vi "HMP_Open_v1.vi"(11 "HMP VISA":refnum<visa-resource-name>="HMP") -> (3 "HMP VISA Out":refnum<visa-resource-name>)   [LabVIEW 2019]
panel:
  out "Loop Error?":errorcluster
  in  "stop":bool
  out "Instructional Message":string
  out "Unsuccesful Attempts to connect":i32
  in  "Error In":errorcluster caption="error in (no error)"
  out "Error Out":errorcluster caption="error out"
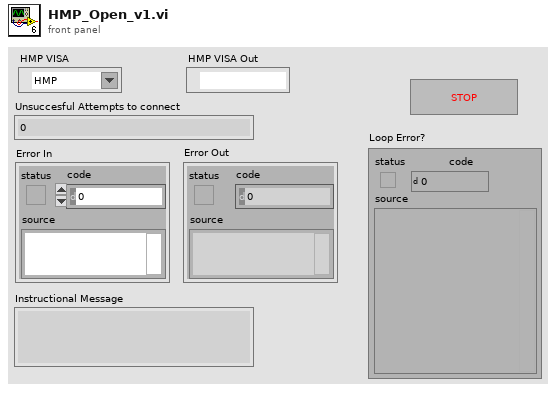
[diagram p1: front panel]
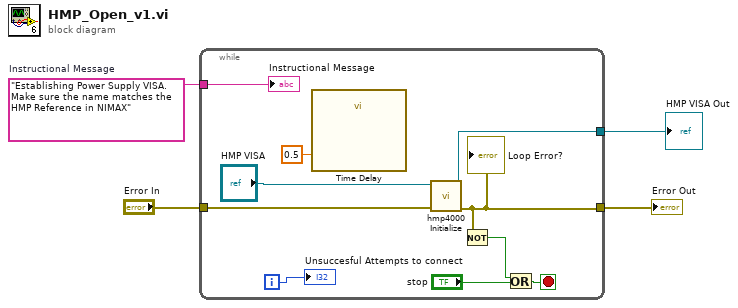
[diagram p0: block diagram]
diagram:
  w2 = "Establishing Power Supply VISA. Make sure the name matches the HMP Reference in NIMAX"  # Instructional Message
  n1 = while {
    tunnel: "Error In" -> [w14]
    tunnel: [w11] -> w4
    tunnel: w2 -> [w9]
    tunnel: [w7] -> w1
    i -> [w8]
    stop <- w10 stop-if-true
    n2 = call "Time Delay"("Delay Time (s)"=0.5) -> ()  [unwired: 10 in, 1 out]
    n3 = call <instrlib>:"hmp4000 Initialize.vi"("error in (no error)"=w14, "VISA resource name"="HMP VISA") -> ("error out"=w11:errorcluster, "VISA resource name out"=w7:refnum<visa-resource-name>)  [unwired: 8 in]
    "Loop Error?" <- w11
    n4 = Not(x=w11) -> (.not. x?=w12:bool)
    n5 = Or(x=w12, y="stop") -> (x .or. y?=w10:bool)
    "Instructional Message" <- w9
    "Unsuccesful Attempts to connect" <- w8
  }
  "Error Out" <- w4
  "HMP VISA Out" <- w1
